vi "FormatTime String.vi"(1 "Numeric":dbl=60.0 format="%0.2f") -> (0 "Date/Time":string="00:01:00")   [LabVIEW 2013]
panel:
  out "Days":dbl format="%0.2f"
  out "Hours":dbl format="%0.2f"
  out "Minutes":dbl=1.0 format="%0.2f"
  out "Seconds":dbl format="%0.2f"
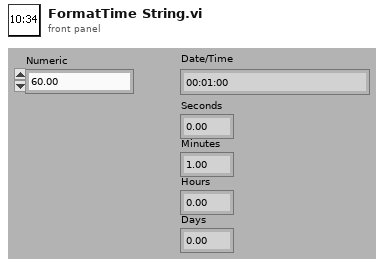
[diagram p1: front panel]
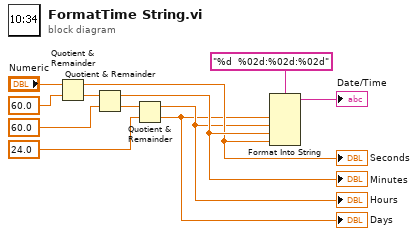
[diagram p0: block diagram]
diagram:
  n1 = Quotient & Remainder(x="Numeric", y=60.0) -> (x-y*floor(x/y)=w5:dbl, floor(x/y)=w10:dbl)
  "Seconds" <- w5
  n2 = Quotient & Remainder(x=w10, y=60.0) -> (x-y*floor(x/y)=w7:dbl, floor(x/y)=w3:dbl)
  "Minutes" <- w7
  n3 = Quotient & Remainder(x=w3, y=24.0) -> (x-y*floor(x/y)=w2:dbl, floor(x/y)=w1:dbl)
  "Hours" <- w2
  "Days" <- w1
  n4 = Format Into String(format string="%d  %02d:%02d:%02d" ("Format String"), w1, w2, w7, w5) -> (resulting string=→"Date/Time":string)  [unwired: 2 in, 1 out]
